vi "simx Start.vi"(5 "commThreadCycleInMs":i32, 6 "timeOutInMs":i32, 7 "doNotReconnectOnceDisconnected":u8, 8 "error in (no error)":errorcluster, 9 "waitUntilConnected":u8, 10 "connectionPort":i32, 11 "connectionAddress":string) -> (0 "error out":errorcluster, 3 "function return":i32)   [LabVIEW 2019, in "PXL_V-REP.lvlib"]
doc: "EXTAPI_DLLEXPORT simxInt simxStart(const simxChar* connectionAddress,simxInt connectionPort,simxUChar waitUntilConnected,simxUChar doNotReconnectOnceDisconnected,simxInt timeOutInMs,simxInt commThreadCycleInMs);"
uses:
  PXL_V-REP.lvlib
  <userlib>/V-REP/remoteApi.dll
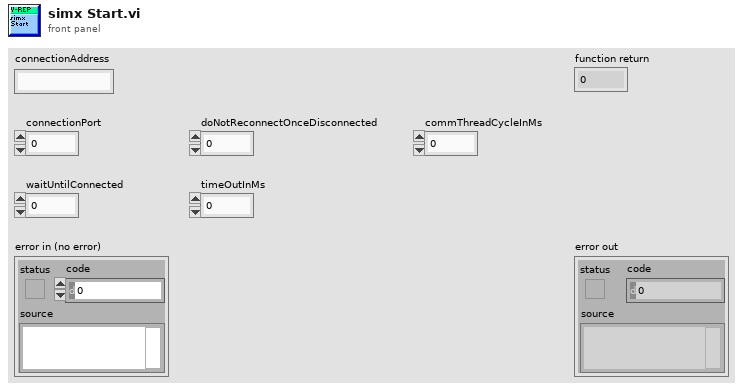
[diagram p1: front panel]
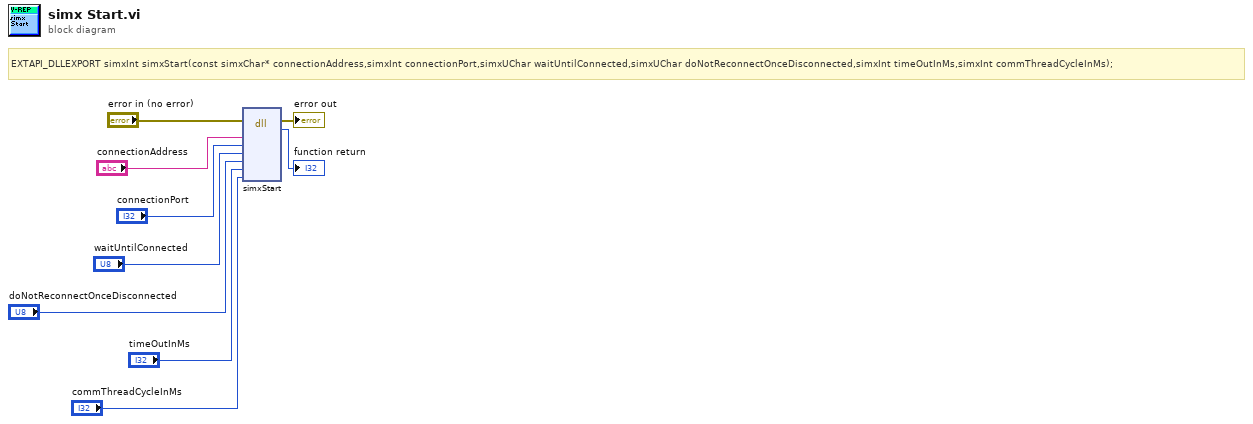
[diagram p0: block diagram]
diagram:
  # "EXTAPI_DLLEXPORT simxInt simxStart(const simxChar* connectionAddress,simxInt connectionPort,simxUChar waitUntilConnected,simxUChar doNotReconnectOnceDisconnected,simxInt timeOutInMs,simxInt commThreadCycleInMs);"
  n1 = dll-call lib="C:/Program Files (x86)/National Instruments/LabVIEW 2019/user.lib/V-REP/remoteApi.*" fn="simxStart"(error in="error in (no error)", "connectionAddress"="connectionAddress", "connectionPort"="connectionPort", "waitUntilConnected"="waitUntilConnected", "doNotReconnectOnceDisconnected"="doNotReconnectOnceDisconnected", "timeOutInMs"="timeOutInMs", "commThreadCycleInMs"="commThreadCycleInMs") -> (error out=→"error out":errorcluster, →"function return":i32)  [unwired: 8 in, 1 out]
